vi "rqcBob ServiceNET Send Command.vi"(8 "error in":errorcluster, 10 "command":T1, 11 "rqcBob ServiceNET in":T2) -> (0 "error out":errorcluster, 3 "rqcBob ServiceNET out":T2)   [LabVIEW 2018]
uses:
  Custom Controls/rqcBob ServiceNET control.ctl
  Custom Controls/rqc ServiceNET command.ctl
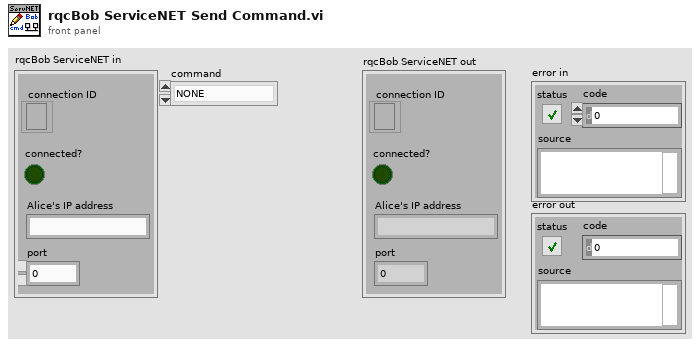
[diagram p1: front panel]
types:
  T1 = typedef "rqc ServiceNET command.ctl" = enum8{"NONE", "READY", "START", "PING"}
  T2 = typedef "rqcBob ServiceNET control.ctl" = cluster{"connection ID":refnum<k5>, "connected?":bool, "Alice's IP address":string, "port":u16}
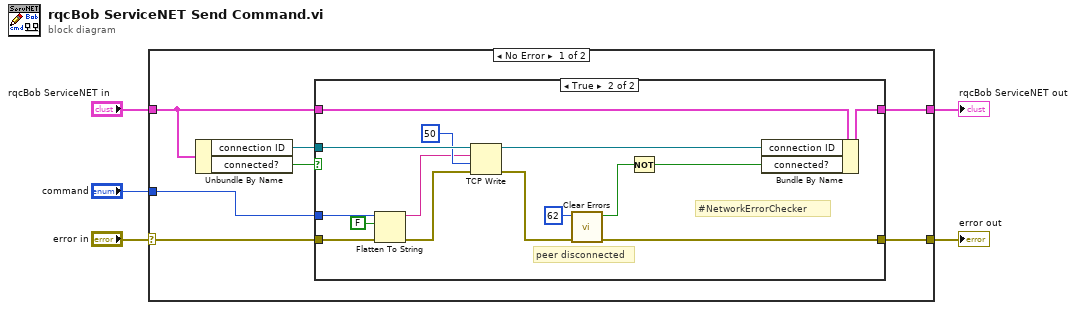
[diagram p0: block diagram]
diagram:
  n1 = case shown="No Error" "error in" {
    selector: "error in" -> [w9 w31]
    tunnel: "rqcBob ServiceNET in" -> [w7 w30]
    tunnel: [w8 w31] -> w3
    tunnel: [w6 w30] -> w2
    tunnel: "command" -> [w10 _]
    frame No Error {
      n2 = Unbundle By Name(w7) -> ("connection ID"=w11:refnum<k5>, "connected?"=w12:bool)
      n3 = case shown="True" w12 {
        tunnel: w11 -> [_ w29]
        tunnel: w10 -> [_ w28]
        tunnel: w9 -> [w14 w27]
        tunnel: [w14 w18] -> w8
        tunnel: [w13 w24] -> w6
        tunnel: w7 -> [w13 w25]
        frame False {
        }
        frame True {
          # "peer disconnected"
          # "#NetworkErrorChecker"
          n4 = Flatten To String(anything=w28, prepend array or string size? (T)=FALSE, error in (no error)=w27) -> (data string=w22:string, error out=w20:errorcluster)  [unwired: 1 in, 1 out]
          n5 = TCP Write(connection ID=w29, data in=w22, error in (no error)=w20, 9:50 ("timeout ms (25000)")) -> (connection ID out=w21:refnum<k5>, error out=w19:errorcluster)  [unwired: 1 out]
          n6 = call <vilib>:"Clear Errors.vi"("error in (no error)"=w19, "specific error code to clear (0: all)"=62) -> ("error out"=w18:errorcluster, "specific error cleared?"=w16:bool)  [unwired: 4 in]
          n7 = Not(x=w16) -> (.not. x?=w15:bool)
          n8 = Bundle By Name(cluster=w25, "connection ID"=w21, "connected?"=w15) -> (w24:T2)
        }
      }
    }
    frame Error {
    }
  }
  "error out" <- w3
  "rqcBob ServiceNET out" <- w2
